vi "TestExec.Control, Remote Launch Test.vi"(6 "Sequence":string, 7 "Module Q Name":string, 8 "error in":errorcluster, 9 "Position":string, 10 "SN":string, 11 "Q In":refnum<queue>) -> (0 "error out":errorcluster)   [LabVIEW 2018]
uses:
  <vilib>/KATE/Queues/Q.Element.ctl
  TestExec.Test Launch Params.ctl
  <vilib>/KATE/Queues/Queue Utils.lvlib
panel:
  out "Q Out":refnum<queue>
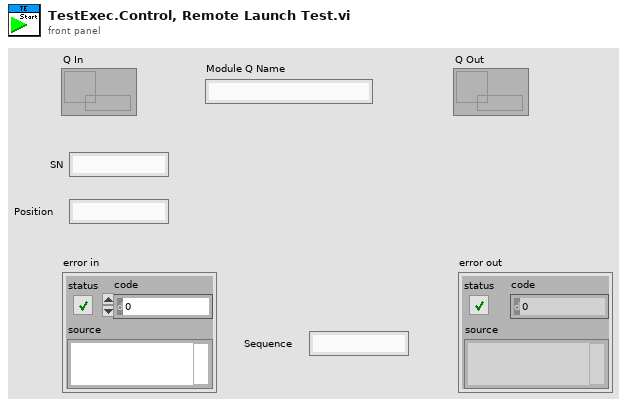
[diagram p1: front panel]
types:
  T1 = typedef "TestExec.Test Launch Params.ctl" = cluster{"Sequence":string, "SN":string, "Pos":string}
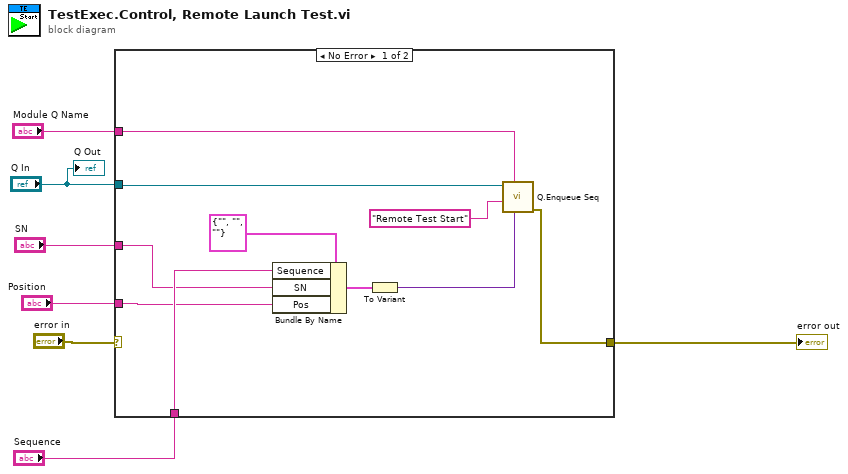
[diagram p0: block diagram]
diagram:
  n1 = case shown="No Error" "error in" {
    selector: "error in" -> [_ w18]
    tunnel: [w16 w18] -> w6
    tunnel: "Q In" -> [w8 _]
    tunnel: "Module Q Name" -> [w15 _]
    tunnel: "SN" -> [w12 _]
    tunnel: "Position" -> [w11 _]
    tunnel: "Sequence" -> [w13 _]
    frame No Error {
      n2 = Bundle By Name(cluster=T1 {"Sequence"="", "SN"="", "Pos"=""}, "Sequence"=w13, "SN"=w12, "Pos"=w11) -> (w10:T1)
      n3 = To Variant(anything=w10) -> (Variant=w9:variant)
      n4 = call <vilib>:"Q.Enqueue Seq.vi"("Data1"=w9, "Q Name"=w15, "Seq Task Name"="Remote Test Start", "Q In"=w8) -> ("error out"=w16:errorcluster)  [unwired: 6 in, 1 out]
    }
    frame Error {
    }
  }
  "error out" <- w6
  "Q Out" <- "Q In"
